vi "FGV_Timestamps_Task.vi"(8 "error in":errorcluster, 10 "Action":T1, 11 "CTR Timestamps  task IN":refnum<k21>) -> (0 "error out":errorcluster, 3 "CTR Timestamps task OUT":refnum<k21>)   [LabVIEW 2026]
doc: "Functional Global Variable:\n- Write the value into the memory \nor\n- Read the value from the memory"
uses:
  controls/TypeDef_FGV.ctl
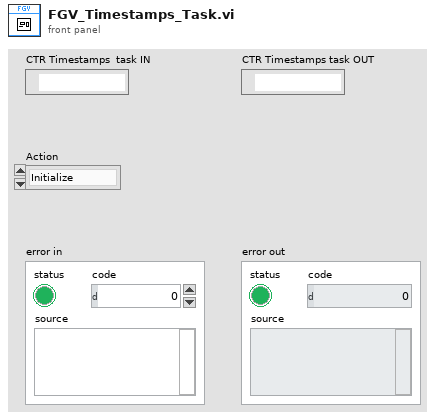
[diagram p1: front panel]
types:
  T1 = typedef "TypeDef_FGV.ctl" = enum16{"Initialize", "Add", "Read"}
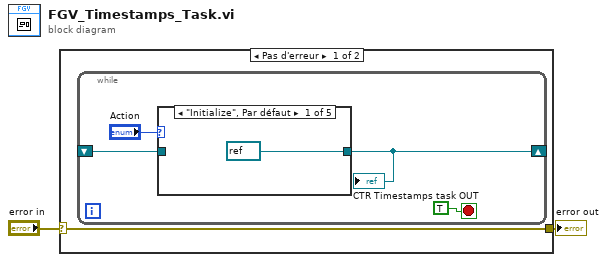
[diagram p0: block diagram]
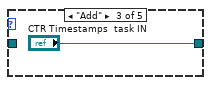
[diagram p3: hidden frame]
diagram:
  n1 = case shown="Pas d'erreur" "error in" {
    selector: "error in" -> [w3 w13]
    tunnel: [w3 w13] -> w1
    frame No Error {
      n2 = while {
        shift-right: [w4] -> _
        shift-left: _ -> [w5]
        stop <- TRUE stop-if-true
        n3 = case shown="\"Initialize\", Par défaut" "Action" {
          tunnel: w5 -> [_ w9 _ w11 w12]
          tunnel: [refnum<k21> refnum ("task out") w9 "CTR Timestamps  task IN" w11 w12] -> w4
          frame "Initialize", Default {
          }
          frame "Read" {
          }
          frame "Add" {
          }
          frame "Initialize" {
            # "A FAIRE"
          }
          frame "Read" {
            # "A Faire"
          }
        }
        "CTR Timestamps task OUT" <- w4
      }
    }
    frame Error {
    }
  }
  "error out" <- w1
